vi "Parse String to Array_String.vi"(6 "Spliter 2":string, 11 "String Input":string) -> (2 "Data 2":string[][](array[string]), 3 "Data 1":string[](array[string]))   [LabVIEW 2020, in "GUCalibration2.lvlib"]
uses:
  GUCalibration2.lvlib
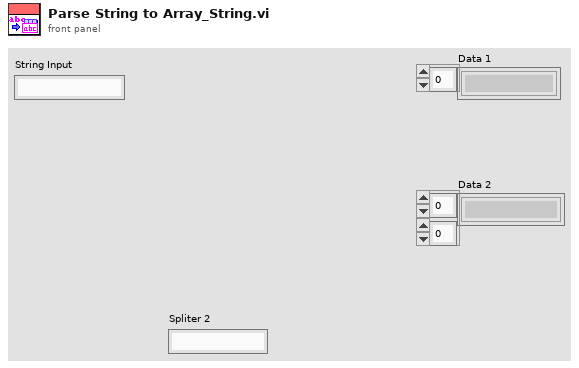
[diagram p1: front panel]
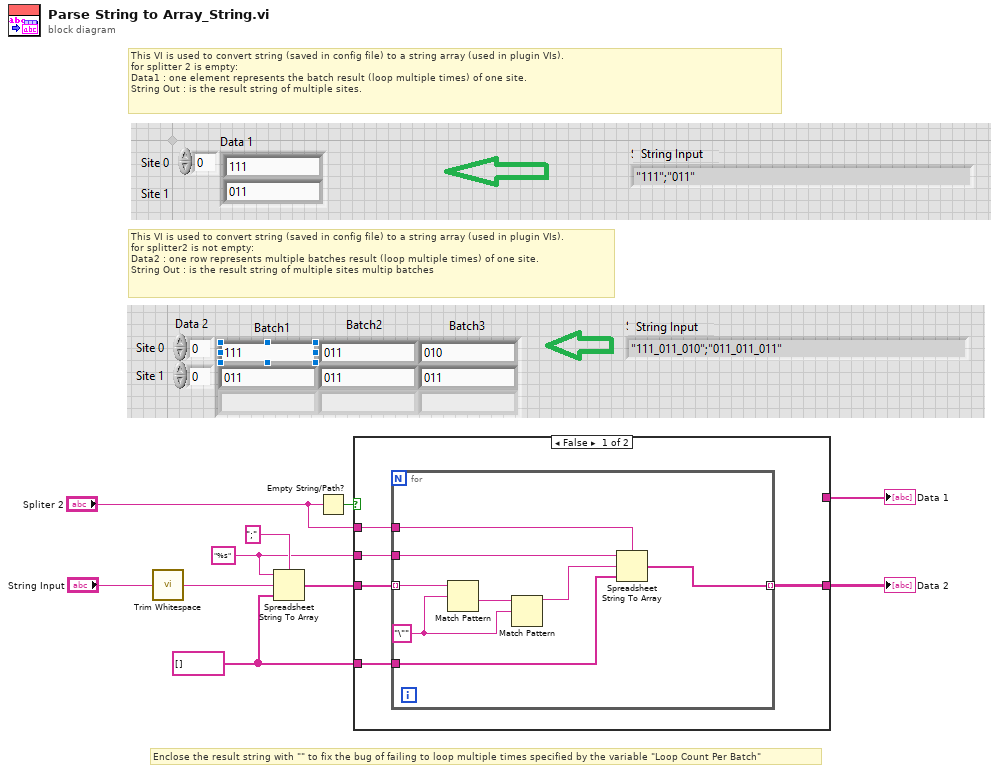
[diagram p0: block diagram]
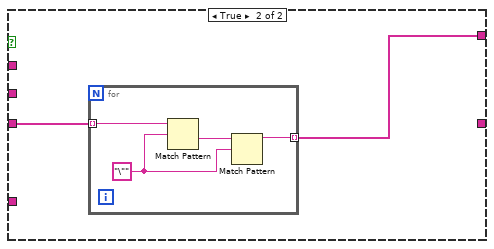
[diagram p2: hidden frame]
diagram:
  w1 = "%s" ("format string")
  w3 = string[] []
  # "This VI is used to convert string (saved in config file) to a string array (used in plugin VIs).\nfor splitter2 is not empty:\nData2 : one row represents multiple batches result (loop multiple times) of one site.\nString Out : is the result string of multiple sites multip batches"
  # "This VI is used to convert string (saved in config file) to a string array (used in plugin VIs).\nfor splitter 2 is empty:\nData1 : one element represents the batch result (loop multiple times) of one site.\nString Out : is the result string of multiple sites."
  # "Enclose the result string with \"\" to fix the bug of failing to loop multiple times specified by the variable \"Loop Count Per Batch\""
  n1 = call <vilib>:"Trim Whitespace.vi"("string"="String Input") -> ("trimmed string"=w2:string)  [unwired: 1 in]
  n2 = Spreadsheet String To Array(delimiter (Tab)=";" ("Spliter 1"), format string=w1, spreadsheet string=w2, array type (2D Dbl)=w3) -> (array=w4:string[])
  n3 = Empty String/Path?(string/path="Spliter 2") -> (empty?=w5:bool)
  n4 = case shown="False" w5 {
    tunnel: w4 -> [w15 w25]
    tunnel: "Spliter 2" -> [w11 _]
    tunnel: w3 -> [w14 _]
    tunnel: w1 -> [w13 _]
    tunnel: [w12 _] -> w7
    tunnel: [_ w24] -> w6
    frame False {
      n5 = for {
        tunnel: w15 -> [w19] mode=indexing
        tunnel: w11 -> [w22]
        tunnel: w14 -> [w23]
        tunnel: w13 -> [w21]
        tunnel: [w20] -> w12 mode=indexing
        w17 = "\"" ("regular expression")
        n6 = Match Pattern(string=w19, regular expression=w17) -> (after substring=w18:string)  [unwired: 1 in, 3 out]
        n7 = Match Pattern(string=w18, regular expression=w17) -> (before substring=w16:string)  [unwired: 1 in, 3 out]
        n8 = Spreadsheet String To Array(delimiter (Tab)=w22, format string=w21, spreadsheet string=w16, array type (2D Dbl)=w23) -> (array=w20:string[])
      }
    }
    frame True {
      n9 = for {
        tunnel: w25 -> [w27] mode=indexing
        tunnel: [w26] -> w24 mode=indexing
        w28 = "\"" ("regular expression")
        n10 = Match Pattern(string=w27, regular expression=w28) -> (after substring=w29:string)  [unwired: 1 in, 3 out]
        n11 = Match Pattern(string=w29, regular expression=w28) -> (before substring=w26:string)  [unwired: 1 in, 3 out]
      }
    }
  }
  "Data 2" <- w7
  "Data 1" <- w6
